vi "ReadPortsHeader.vi"(0 "data":string) -> (1 "Numbers":i32[](array[numeric]), 2 "Names":string[](array[string]))   [LabVIEW 2012]
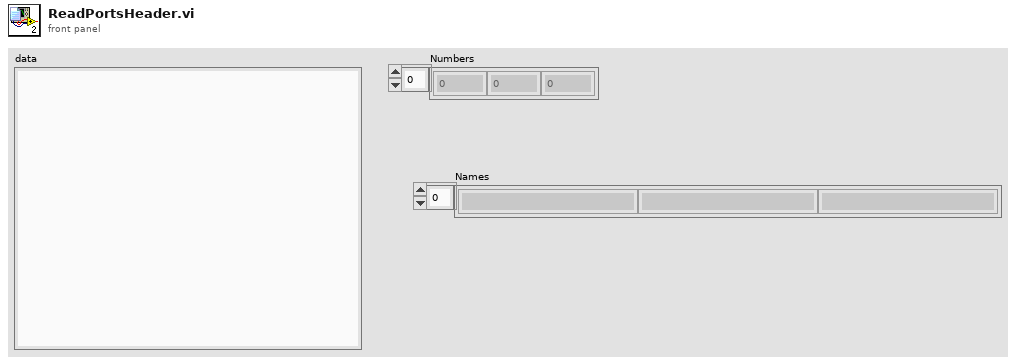
[diagram p1: front panel]
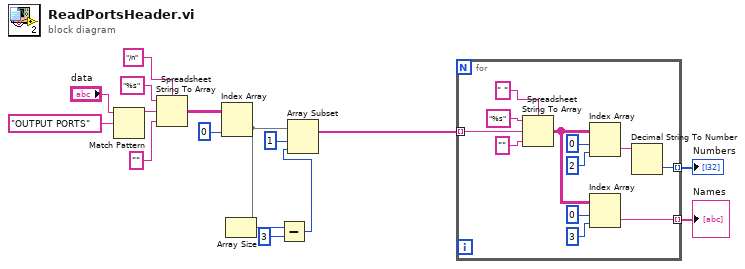
[diagram p0: block diagram]
diagram:
  n1 = Match Pattern(string="data", regular expression="OUTPUT PORTS") -> (before substring=w12:string)  [unwired: 1 in, 3 out]
  n2 = Spreadsheet String To Array(delimiter (Tab)="/n", format string="%s", spreadsheet string=w12, array type (2D Dbl)="" ("delimiter (Tab)")) -> (array=w10:string[][])
  n3 = Index Array(array=w10, index (col)=0 ("index (row)")) -> (element=w4:string[])  [unwired: 1 in]
  n4 = Array Size(array=w4) -> (size(s)=w3:i32)
  n5 = Subtract(x=w3, y=3) -> (x-y=w2:i32)
  n6 = Array Subset(array=w4, index=1, length=w2) -> (w7:string[])
  n7 = for {
    tunnel: w7 -> [w25] mode=indexing
    tunnel: [w21] -> w6 mode=indexing
    tunnel: [w17] -> w5 mode=indexing
    n8 = Spreadsheet String To Array(delimiter (Tab)=" ", format string="%s", spreadsheet string=w25, array type (2D Dbl)="" ("delimiter (Tab)")) -> (array=w18:string[][])
    n9 = Index Array(array=w18, index (row)=0, index (col)=2 ("disabled index (col)")) -> (element=w22:string)
    n10 = Index Array(array=w18, index (row)=0, index (col)=3 ("disabled index (col)")) -> (element=w17:string)
    n11 = Decimal String To Number(string=w22) -> (number=w21:i32)  [unwired: 2 in, 1 out]
  }
  "Numbers" <- w6
  "Names" <- w5
